vi "AES Encrypt.vi"   [LabVIEW 2021, in "dotNET Crypto Symmetric Encryption.lvlib"]
doc: "Encrypt data using AES encryption. ECB and CBC block cipher modes are supported. ECB is considered cryptographically insecure and should not be used."
uses:
  dotNET Crypto Symmetric Encryption.lvlib
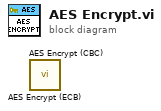
[diagram p0: block diagram]
diagram:
  n1 = call "AES Encrypt (ECB).vi"() -> ()  [unwired: 10 in, 2 out]
  n2 = call "AES Encrypt (CBC).vi"() -> ()  [unwired: 9 in, 3 out]
